vi "cal struct thing.vi"() -> ()   [LabVIEW 2013]
panel:
  out "unsigned byte array":u8[](array[numeric])
  out "CalData 2":T1
  in  "string":string
  out "CalData":T1
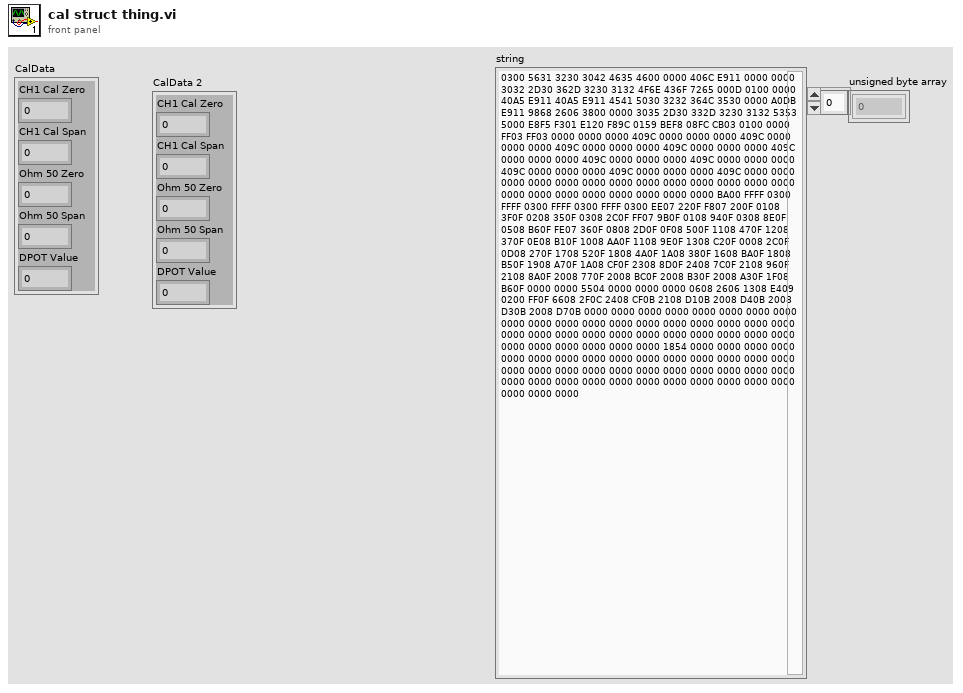
[diagram p1: front panel]
types:
  T1 = cluster{"CH1 Cal Zero ":u32, "CH1 Cal Span":u32, "Ohm 50 Zero ":u32, "Ohm 50 Span ":u32, "DPOT Value ":u32}
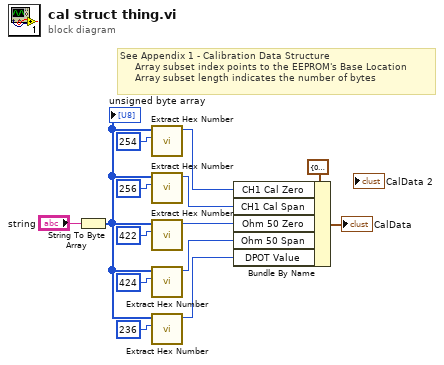
[diagram p0: block diagram]
diagram:
  # "See Appendix 1 - Calibration Data Structure\n     Array subset index points to the EEPROM's Base Location\n     Array subset length indicates the number of bytes"
  n1 = String To Byte Array(string="string") -> (unsigned byte array=w9:u8[])
  "unsigned byte array" <- w9
  n2 = call "Extract Hex Number.vi"("index"=254, "unsigned byte array"=w9) -> ("Numeric"=w10:u16)  [unwired: 9 in]
  n3 = call "Extract Hex Number.vi"("index"=256, "unsigned byte array"=w9) -> ("Numeric"=w8:u16)  [unwired: 9 in]
  n4 = call "Extract Hex Number.vi"("index"=422, "unsigned byte array"=w9) -> ("Numeric"=w7:u16)  [unwired: 9 in]
  n5 = call "Extract Hex Number.vi"("index"=424, "unsigned byte array"=w9) -> ("Numeric"=w6:u16)  [unwired: 9 in]
  n6 = call "Extract Hex Number.vi"("index"=236, "unsigned byte array"=w9) -> ("Numeric"=w5:u16)  [unwired: 9 in]
  n7 = Bundle By Name(cluster=T1 {"CH1 Cal Zero "=0, "CH1 Cal Span"=0, "Ohm 50 Zero "=0, "Ohm 50 Span "=0, "DPOT Value "=0} ("CalstructView"), "CH1 Cal Zero"=w10, "CH1 Cal Span"=w8, "Ohm 50 Zero"=w7, "Ohm 50 Span"=w6, "DPOT Value"=w5) -> (→"CalData":T1)
